vi "S2C_M2p5942_Proc_Status.vi"(8 "Error In":errorcluster) -> (0 "Error Out":errorcluster, 3 "Response":string)   [LabVIEW 2024]
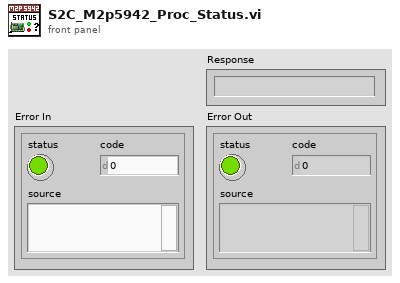
[diagram p1: front panel]
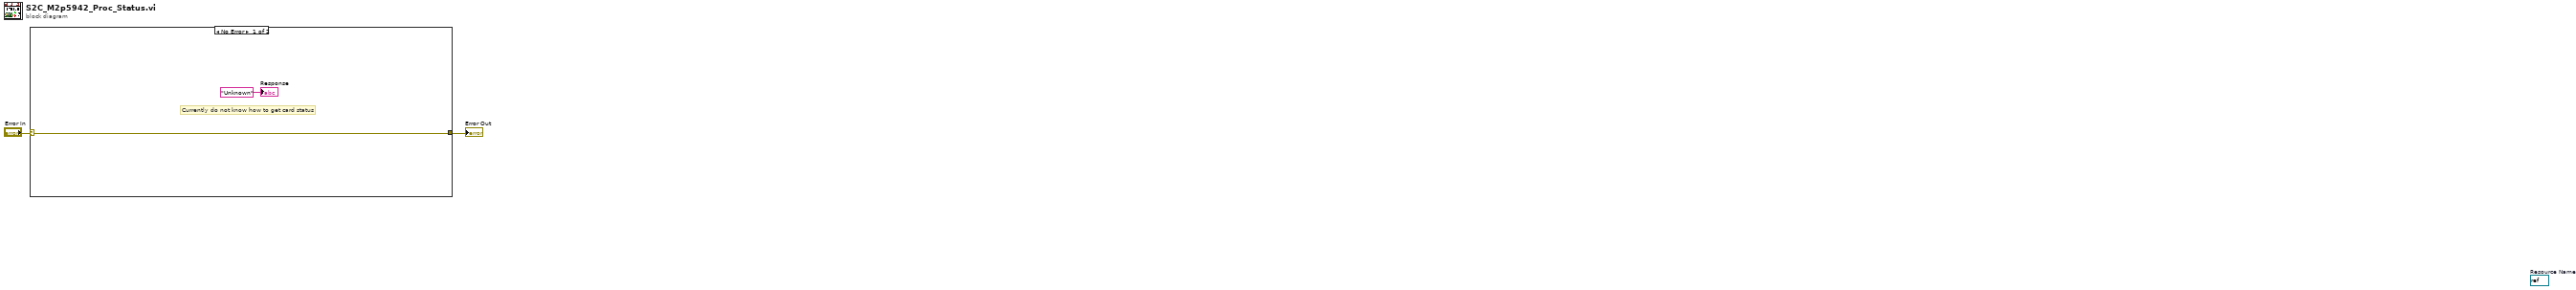
[diagram p0: block diagram]
diagram:
  (unwired) refnum<visa-resource-name> refnum  # Resource Name
  n1 = case shown="No Error" "Error In" {
    selector: "Error In" -> [w4 w5]
    tunnel: [w4 w5] -> w1
    frame No Error {
      # "Currently do not know how to get card status"
      "Response" <- "Unknown" ("Response")
    }
    frame Error {
    }
  }
  "Error Out" <- w1
